vi "FlipARGB.vi"(7 "Flip Mode (Default: Y-Axis)":T1=enum."Y-Axis", 8 "error in (no error)":errorcluster, 10 "ARGB Destination Image":refnum<data-value>, 11 "ARGB Source Image":refnum<data-value>) -> (0 "error out":errorcluster, 3 "ARGB  Destination Image (duplicate)":refnum<data-value>)   [LabVIEW 2020, in "g_ar_toolkit.image.lvlib"]
uses:
  g_ar_toolkit.image.lvlib
  Flip Mode.ctl
  <vilib>/Utility/error.llb/Error Cluster From Error Code.vi
  348de330-10c9-445f-8d54-7780e9118077.vi
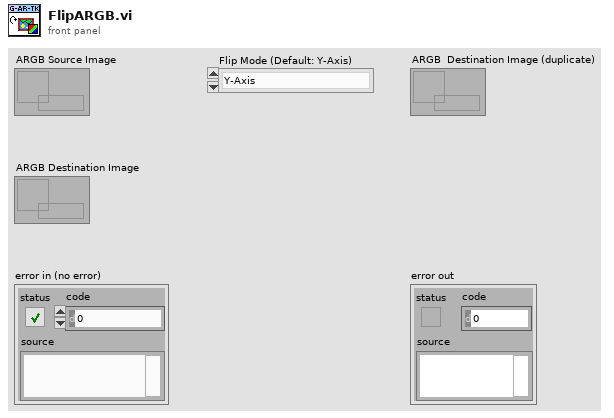
[diagram p1: front panel]
types:
  T1 = typedef "g_ar_toolkit.image.lvlib/Flip Mode.ctl" = enum8{"X-Axis", "Y-Axis", "X and Y Axes"}
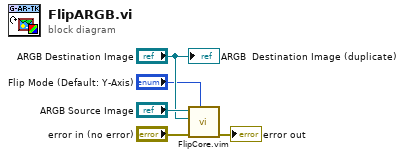
[diagram p0: block diagram]
diagram:
  n1 = call "FlipCore.vim"("Flip Mode"="Flip Mode (Default: Y-Axis)", "error in (no error)"="error in (no error)", "Destination Image"="ARGB Destination Image", "Source Image"="ARGB Source Image") -> ("error out"=→"error out":errorcluster)  [unwired: 7 in]
  "ARGB  Destination Image (duplicate)" <- "ARGB Destination Image"
